vi "Write status.vi"(8 "error in (no error)":errorcluster, 10 "Status":i32, 11 "PV in":refnum<class "PV.lvclass">) -> (0 "error out":errorcluster, 3 "PV out":refnum<class "PV.lvclass">)   [LabVIEW 2016, in "CS++ProcessVariables.lvlib" / "PV.lvclass"]
doc: "Write Status."
uses:
  PV.lvclass
  PV.lvclass/PV.ctl
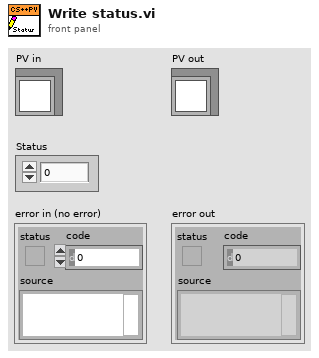
[diagram p1: front panel]
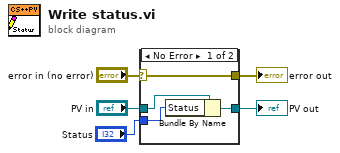
[diagram p0: block diagram]
diagram:
  n1 = case shown="No Error" "error in (no error)" {
    selector: "error in (no error)" -> [w9 w10]
    tunnel: [w9 w10] -> w4
    tunnel: [w7 w11] -> w2
    tunnel: "PV in" -> [w8 w11]
    tunnel: "Status" -> [w6 _]
    frame No Error {
      n2 = Bundle By Name(cluster=w8, "Status"=w6) -> (w7:refnum<class "PV.lvclass">)
    }
    frame Error {
    }
  }
  "error out" <- w4
  "PV out" <- w2
